vi "Pemula 5.vi"() -> ()   [LabVIEW 2017]
panel:
  in  "Save Button":bool
  in  "Home Button":bool
  out "Waveform Chart":cluster{dbl, dbl, dbl}(graph)
  out "Table Control":string[][](table)
  in  "Play Button":bool
  in  "stop":bool
  out "s? t:f":string
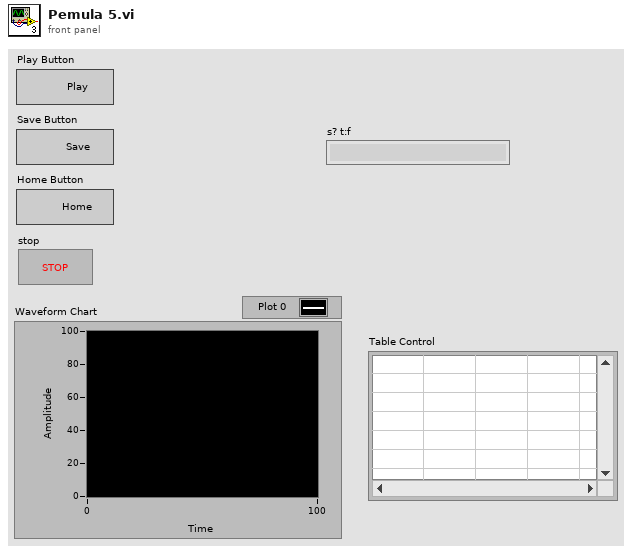
[diagram p1: front panel]
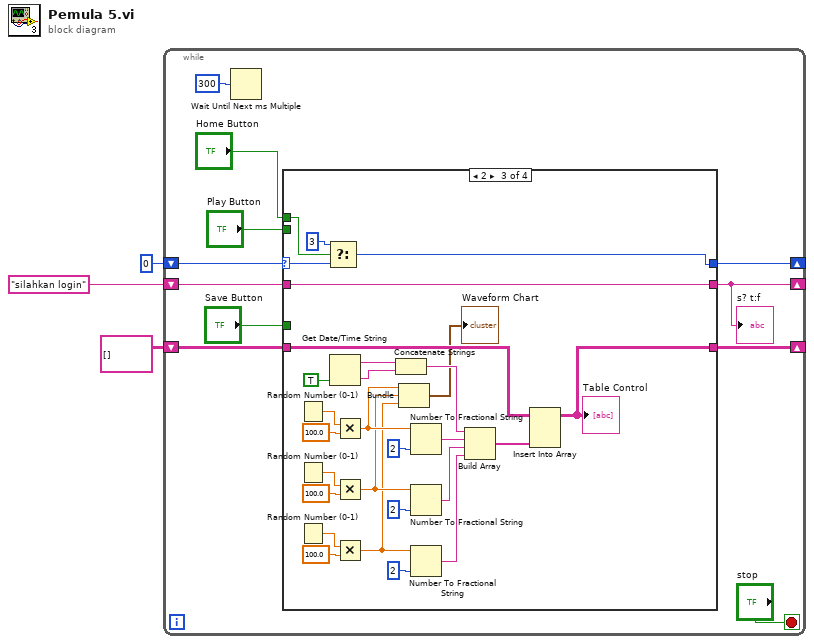
[diagram p0: block diagram]
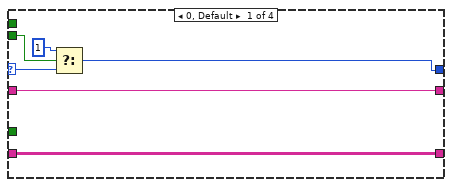
[diagram p2: hidden frame]
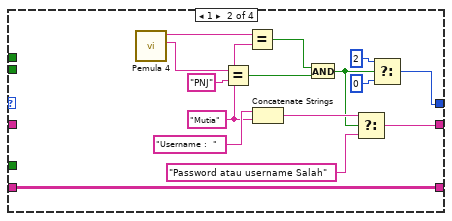
[diagram p3: hidden frame]
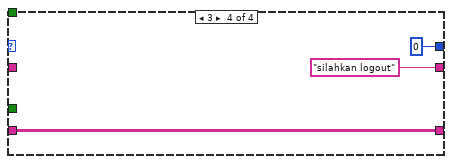
[diagram p4: hidden frame]
diagram:
  n1 = while {
    shift-right: [w13] -> _
    shift-left: 0 -> [w14]
    shift-right: [w9] -> _
    shift-left: string[][] [] -> [w10]
    shift-right: [w7] -> _
    shift-left: "silahkan login" ("f") -> [w6]
    stop <- "stop" stop-if-true
    n2 = Wait Until Next ms Multiple(millisecond multiple=u32 300) -> ()  [unwired: 1 out]
    n3 = case shown="2" w14 {
      selector: w14 -> [w16 _ w38 _]
      tunnel: "Play Button" -> [w20 _ _ _]
      tunnel: [w18 w23 w37 0] -> w13
      tunnel: w10 -> [w17 w22 w48 w64]
      tunnel: [w17 w22 w42 w64] -> w9
      tunnel: [w15 w21 w41 "silahkan logout" ("f")] -> w7
      tunnel: "Home Button" -> [_ _ w40 _]
      tunnel: w6 -> [w15 _ w41 _]
      tunnel: "Save Button" -> [_ _ _ _]
      frame 0, Default {
        n4 = Select(t=1, s=w20, f=w16) -> (s? t:f=w18:i32)
      }
      frame 1 {
        w29 = "Mutia" ("y")
        n5 = call "Pemula 4.vi"() -> ("Password 2"=w33:string, "Username 2"=w35:string)  [unwired: 8 in, 1 out]
        n6 = Equal?(x=w33, y="PNJ") -> (x = y?=w31:bool)
        n7 = Equal?(x=w35, y=w29) -> (x = y?=w32:bool)
        n8 = Concatenate Strings("Username :  " ("y"), w29) -> (w28:string)
        n9 = And(x=w32, y=w31) -> (x .and. y?=w26:bool)
        n10 = Select(t=w28, s=w26, f="Password atau username Salah") -> (s? t:f=w21:string)
        n11 = Select(t=2, s=w26, f=0) -> (s? t:f=w23:i32)
      }
      frame 2 {
        n12 = Random Number (0-1)() -> (number: 0 to 1=w58:dbl)
        n13 = Random Number (0-1)() -> (number: 0 to 1=w57:dbl)
        n14 = Random Number (0-1)() -> (number: 0 to 1=w56:dbl)
        n15 = Select(t=3, s=w40, f=w38) -> (s? t:f=w37:i32)
        n16 = Get Date/Time String(want seconds? (F)=TRUE) -> (date string=w60:string, time string=w59:string)  [unwired: 2 in]
        n17 = Multiply(x=w58, y=100.0) -> (x*y=w45:dbl)
        n18 = Multiply(x=w57, y=100.0) -> (x*y=w44:dbl)
        n19 = Multiply(x=w56, y=100.0) -> (x*y=w36:dbl)
        n20 = Concatenate Strings(w60, w59) -> (w55:string)
        n21 = Bundle(w45, w44, w36) -> (→"Waveform Chart":cluster{dbl, dbl, dbl})  [unwired: 1 in]
        n22 = Number To Fractional String(number=w45, precision (6)=i16 2) -> (F-format string=w51:string)  [unwired: 2 in]
        n23 = Number To Fractional String(number=w44, precision (6)=i16 2) -> (F-format string=w50:string)  [unwired: 2 in]
        n24 = Number To Fractional String(number=w36, precision (6)=i16 2) -> (F-format string=w49:string)  [unwired: 2 in]
        n25 = Build Array(w55, w51, w50, w49) -> (w47:string[])
        n26 = Insert Into Array(array=w48, new element=w47) -> (w42:string[][])  [unwired: 2 in]
        "Table Control" <- w42
      }
      frame 3 {
      }
    }
    "s? t:f" <- w7
  }
